vi "temporary load classes.vi"(8 "error in":errorcluster, 10 "config class path":path, 11 "runtime class path":path) -> (0 "error out":errorcluster, 1 "index ctl":string[](array[string]), 2 "data ctl":string[](array[string]), 3 "valid?":bool[](array[boolean]))   [LabVIEW 2013, in "data interface script.lvlib"]
uses:
  data interface script.lvlib
  module/execution/fixed channel runtime.lvclass
  module/configuration/fixed channel configuration.lvclass
  <vilib>/Utility/VariantDataType/VariantType.lvlib
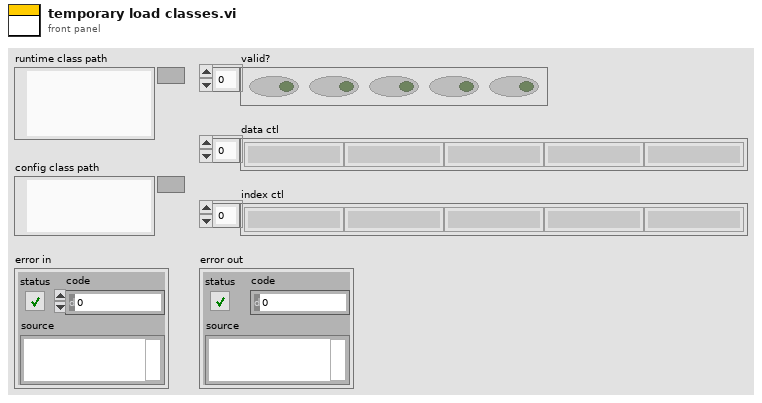
[diagram p1: front panel]
types:
  T1 = typedef "fixed channel runtime.lvclass/data cluster type definition.ctl" = cluster{"input data":variant, "parameter data":variant, "result data":variant, "output data":variant}
  T2 = typedef "fixed channel configuration.lvclass/index type definitions.ctl" = cluster{"input indices":variant, "parameter indices":variant, "result indices":variant, "output indices":variant}
  T3 = typedef "VariantType.lvlib/TypedefInfo.ctl" = cluster{"Name":string, "Timestamp":u32}
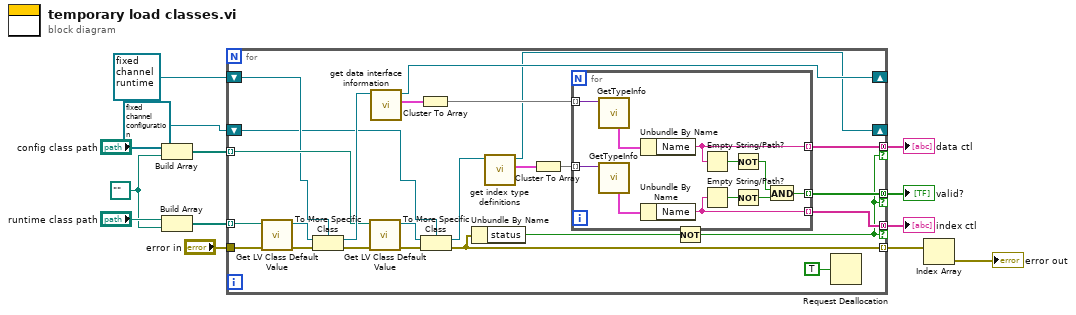
[diagram p0: block diagram]
diagram:
  w3 = path "" ("element")
  n1 = Build Array("config class path", w3) -> (w4:path[])
  n2 = Build Array("runtime class path", w3) -> (w5:path[])
  n3 = for {
    tunnel: [w38] -> w13 mode=concatenating if=w18
    tunnel: [w37] -> w12 mode=concatenating if=w18
    tunnel: [w36] -> w11 mode=concatenating if=w18
    tunnel: w4 -> [w23] mode=indexing
    tunnel: w5 -> [w22] mode=indexing
    tunnel: "error in" -> [w31]
    tunnel: [w20] -> w9 mode=indexing
    shift-right: [w16] -> _
    shift-left: refnum<class "fixed channel runtime.lvclass"> refnum ("fixed channel runtime") -> [w17]
    shift-right: [w14] -> _
    shift-left: refnum<class "fixed channel configuration.lvclass"> refnum ("fixed channel configuration") -> [w15]
    n4 = call <vilib>:"Get LV Class Default Value.vi"("error in (no error)"=w31, "class path"=w22) -> ("error out"=w27:errorcluster, "object"=w26:refnum<class>)  [unwired: 8 in]
    n5 = To More Specific Class(target class=w17, reference=w26, error in=w27) -> (specific class reference=w28:refnum<class "fixed channel runtime.lvclass">, error out=w30:errorcluster)
    n6 = call <vilib>:"Get LV Class Default Value.vi"("error in (no error)"=w30, "class path"=w23) -> ("error out"=w24:errorcluster, "object"=w25:refnum<class>)  [unwired: 8 in]
    n7 = call-dynamic "get data interface information.vi"("fixed channel runtime in"=w28) -> ("data type defs"=w33:T1, "fixed channel runtime out"=w16:refnum<class "fixed channel runtime.lvclass">)  [unwired: 9 in]
    n8 = Cluster To Array(cluster=w33) -> (array=w35:variant[])
    n9 = To More Specific Class(target class=w15, reference=w25, error in=w24) -> (specific class reference=w29:refnum<class "fixed channel configuration.lvclass">, error out=w20:errorcluster)
    n10 = Unbundle By Name(w20) -> ("status"=w19:bool)
    n11 = call-dynamic "get index type definitions.vi"("fixed channel configuration in"=w29) -> ("index type defs"=w32:T2, "fixed channel configuration out"=w14:refnum<class "fixed channel configuration.lvclass">)  [unwired: 9 in]
    n12 = Cluster To Array(cluster=w32) -> (array=w34:variant[])
    n13 = for {
      tunnel: w34 -> [w41] mode=indexing
      tunnel: w35 -> [w44] mode=indexing
      tunnel: [w48] -> w36 mode=indexing
      tunnel: [w45] -> w37 mode=indexing
      tunnel: [w40] -> w38 mode=indexing
      n14 = call <vilib>:"GetTypeInfo.vi"("Variant"=w44) -> ("TypedefInfo"=w49:T3)  [unwired: 6 in, 4 out]
      n15 = call <vilib>:"GetTypeInfo.vi"("Variant"=w41) -> ("TypedefInfo"=w42:T3)  [unwired: 6 in, 4 out]
      n16 = Unbundle By Name(w49) -> ("Name"=w45:string)
      n17 = Unbundle By Name(w42) -> ("Name"=w40:string)
      n18 = Empty String/Path?(string/path=w45) -> (empty?=w46:bool)
      n19 = Empty String/Path?(string/path=w40) -> (empty?=w43:bool)
      n20 = Not(x=w46) -> (.not. x?=w47:bool)
      n21 = Not(x=w43) -> (.not. x?=w39:bool)
      n22 = And(x=w47, y=w39) -> (x .and. y?=w48:bool)
    }
    n23 = Not(x=w19) -> (.not. x?=w18:bool)
    n24 = Request Deallocation(TRUE ("flag")) -> ()
  }
  "index ctl" <- w13
  "data ctl" <- w12
  "valid?" <- w11
  n25 = Index Array(array=w9) -> (element=→"error out":errorcluster)  [unwired: 1 in]
